vi "Driver VI Template Name.vi"(11 "CD Template":refnum<class "NIVS_Inline Model Interface.lvclass">) -> (2 "Driver VI Template Name":string)   [LabVIEW 2015, in "NIVS_Inline Model Interface.lvclass"]
uses:
  NIVS_Inline Model Interface.lvclass
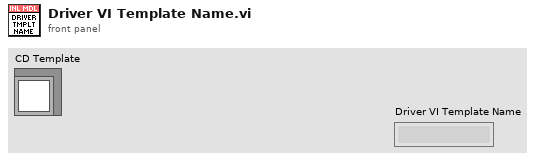
[diagram p1: front panel]
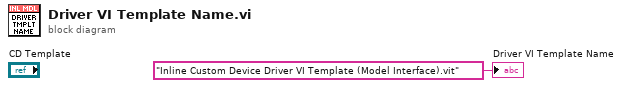
[diagram p0: block diagram]
diagram:
  "Driver VI Template Name" <- "Inline Custom Device Driver VI Template (Model Interface).vit" ("Driver VI Template Name")
